vi "calculator.vi"() -> ()   [LabVIEW 2016]
panel:
  in  "Y":dbl
  in  "X":dbl
  in  "Operation":enum16{"ADD", "SUBTRACT", "MULTIPLY", "DIVIDE"}(ring)
  out "Result":dbl
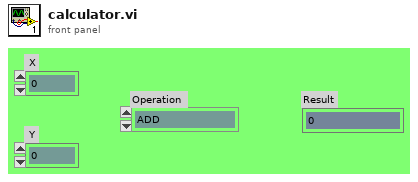
[diagram p1: front panel]
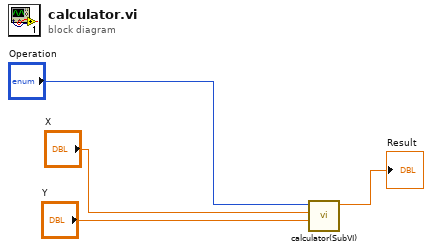
[diagram p0: block diagram]
diagram:
  n1 = call "calculator(SubVI).vi"("Y"="Y", "X"="X", "Operation"="Operation") -> ("Numeric"=→"Result":dbl)  [unwired: 8 in]
